vi "TDS Analog Input Read.vi"(8 "error in (no error)":errorcluster, 10 "Signal InstConfig":string, 11 "Address":string) -> (0 "error out":errorcluster, 3 "Measurement":dbl)   [LabVIEW 2025, in "Interface Functions.lvlib"]
uses:
  Interface Functions.lvlib
panel:
  # "Analog Input Read"
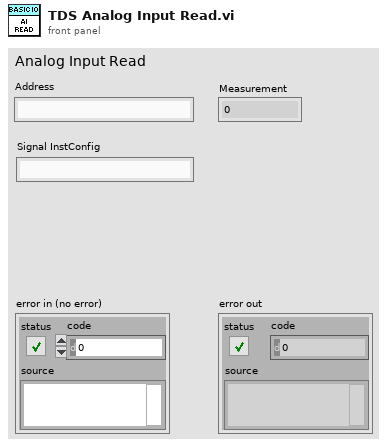
[diagram p1: front panel]
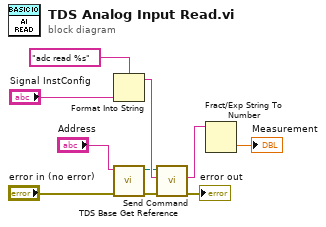
[diagram p0: block diagram]
diagram:
  n1 = Format Into String(format string="adc read %s", "Signal InstConfig") -> (resulting string=w6:string)  [unwired: 2 in, 1 out]
  n2 = call "TDS Base Get Reference.vi"("error in (no error)"="error in (no error)", "Address"="Address") -> ("error out"=w4:errorcluster, "Reference"=w5:refnum<visa-resource-name>)  [unwired: 8 in]
  n3 = call "Send Command.vi"("error in (no error)"=w4, "Command"=w6, "VISA resource name"=w5) -> ("error out"=→"error out":errorcluster, "Read Value"=w2:string)  [unwired: 6 in, 1 out]
  n4 = Fract/Exp String To Number(string=w2) -> (number=→"Measurement":dbl)  [unwired: 3 in, 1 out]
